vi "Parse Sysdef.vi"(0 "Device Reference in":T5 format="%.0x", 5 "error in (no error)":errorcluster) -> (6 "Status Config":T4 {"HWOut Dur Ref" format="%.0x"; "HWIn Dur Ref" format="%.0x"; "Error Data Ref" format="%.0x"}, 10 "HWIn BaseRate":i32, 12 "HWOut BaseRate":i32, 14 "Device Reference out":T5 format="%.0x", 15 "HWOutput Section Data":T6[](array[typedef]) {"Labels Settings"."Label" format="%.0o"}, 17 "HWInput Section Data":T6[](array[typedef]) {"Labels Settings"."Label" format="%.0o"}, 18 "Label Transfer Config":T1 {"Block Data Refs"."Data Reference" format="%.0x"}, 19 "error out":errorcluster)   [LabVIEW 2016, in "Ballard Arinc-429 Engine.lvlib"]
uses:
  Ballard Arinc-429 Engine.lvlib
  RT Controls/RT HW Channel.ctl
  RT Controls/RT Label Settings.ctl
  Shared/Controls and Global/Label.ctl
  Shared/Controls and Global/transferPeriod.ctl
  RT Controls/Driver Data.ctl
  RT Controls/RT Word Settings.ctl
  <vilib>/NI Veristand/Custom Device API/Block Data Reference.ctl
  <vilib>/NI Veristand/Custom Device API/Data Reference.ctl
  RT Controls/RT Param Setting.ctl
  Shared/Controls and Global/Start Bit.ctl
  Shared/Controls and Global/Number of Bits.ctl
  Shared/Controls and Global/TransferType.ctl
  <vilib>/NI Veristand/Custom Device API/Custom Device Item Ref.ctl
  RT Controls/Status Channels Config.ctl
  RT Controls/Label Transfer Config.ctl
  Shared/Controls and Global/Global.vi
  Shared/Ballard Arinc-429 Shared.lvlib
  <vilib>/NI Veristand/Custom Device API/Custom Device API.lvlib
  <vilib>/NI Veristand/Custom Device API/Get Item Property (Boolean).vi
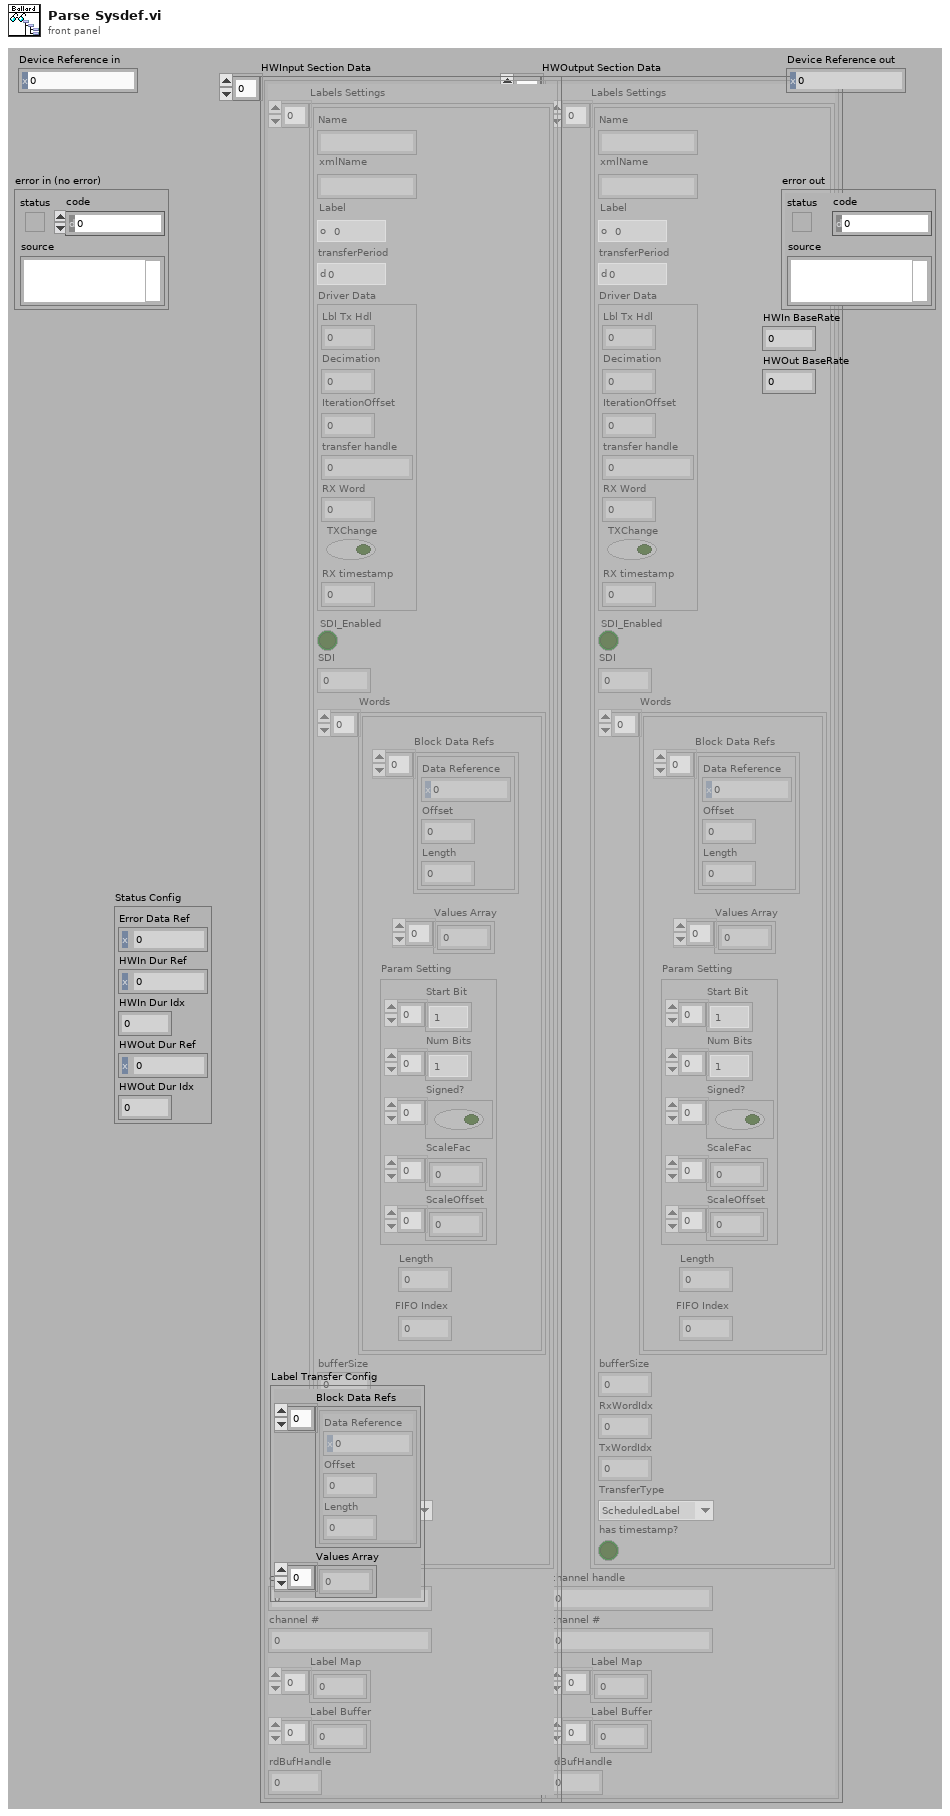
[diagram p1: front panel]
types:
  T1 = typedef "Ballard Arinc-429 Engine.lvlib/Label Transfer Config.ctl" = cluster{"Block Data Refs":T2[], "Values Array":dbl[]}
  T2 = typedef "Custom Device API.lvlib/Block Data Reference.ctl" = cluster{"Data Reference":T3, "Offset":u64, "Length":u64}
  T3 = typedef "Custom Device API.lvlib/Data Reference.ctl" = i32
  T4 = typedef "Ballard Arinc-429 Engine.lvlib/Status Channels Config.ctl" = cluster{"Error Data Ref":T3, "HWIn Dur Ref":T3, "HWIn Dur Idx":i32, "HWOut Dur Ref":T3, "HWOut Dur Idx":i32}
  T5 = typedef "Custom Device API.lvlib/Custom Device Item Ref.ctl" = u64
  T6 = typedef "Ballard Arinc-429 Engine.lvlib/RT HW Channel.ctl" = cluster{"Labels Settings":T7[], "channel handle":u32, "channel #":u16, "Label Map":i32[], "Label Buffer":u32[], "rdBufHandle":u32}
  T7 = typedef "Ballard Arinc-429 Engine.lvlib/RT Label Settings.ctl" = cluster{"Name":string, "xmlName":string, "Label":T8, "transferPeriod":T9, "Driver Data":T10, "SDI_Enabled":bool, "SDI":u8, "Words":T11[], "bufferSize":u32, "RxWordIdx":i32, "TxWordIdx":i32, "TransferType":T15, "has timestamp?":bool}
  T8 = typedef "Ballard Arinc-429 Shared.lvlib/Label.ctl" = u8
  T9 = typedef "Ballard Arinc-429 Shared.lvlib/transferPeriod.ctl" = u32
  T10 = typedef "Ballard Arinc-429 Engine.lvlib/Driver Data.ctl" = cluster{"Lbl Tx Hdl":u32, "Decimation":i32, "IterationOffset":i32, "transfer handle":u32, "RX Word":u32, "TXChange":bool, "RX timestamp":dbl}
  T11 = typedef "Ballard Arinc-429 Engine.lvlib/RT Word Settings.ctl" = cluster{"Block Data Refs":T2[], "Values Array":dbl[], "Length":i32, "FIFO Index":i32, "Param Setting":T12}
  T12 = typedef "Ballard Arinc-429 Engine.lvlib/RT Param Setting.ctl" = cluster{"Start Bit":T13[], "Num Bits":T14[], "Signed?":bool[], "ScaleFac":dbl[], "ScaleOffset":dbl[]}
  T13 = typedef "Ballard Arinc-429 Shared.lvlib/Start Bit.ctl" = i32
  T14 = typedef "Ballard Arinc-429 Shared.lvlib/Number of Bits.ctl" = i32
  T15 = typedef "Ballard Arinc-429 Shared.lvlib/TransferType.ctl" = enum16{"ScheduledLabel", "Acyclic", "Block", "Strobe"}
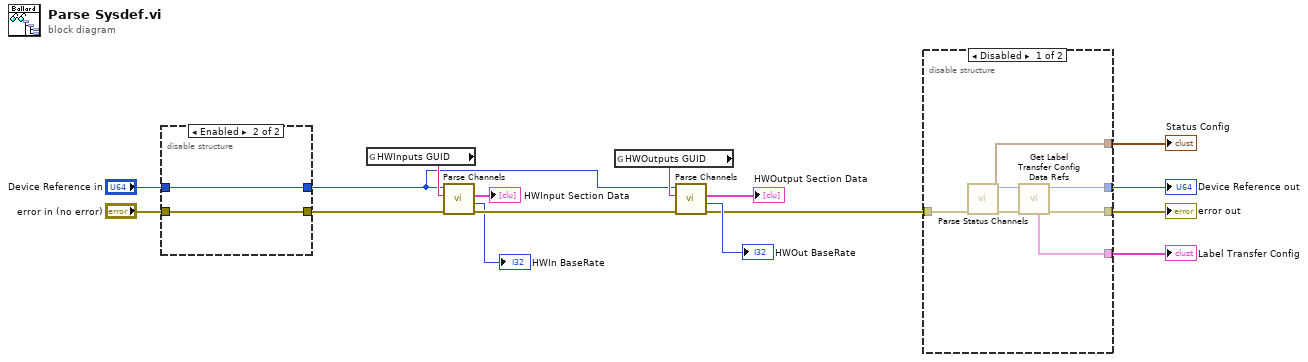
[diagram p0: block diagram]
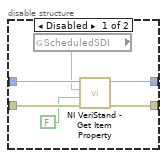
[diagram p3: hidden frame]
diagram:
  n1 = disable-structure shown="Enabled" {
    disable-tunnel: "Device Reference in" -> [w23 w25]
    disable-tunnel: [w22 w25] -> w1
    disable-tunnel: "error in (no error)" -> [w21 w24]
    disable-tunnel: [w20 w24] -> w2
    frame Disabled {
      n2 = global read "Global.vi" "ScheduledSDI"() -> (w18:string)
      n3 = call-poly <vilib>:"NI VeriStand - Get Item Property.vi"("error in (no error)"=w21, "Default Value"=FALSE, "Property Name"=w18, "Item Ref in"=w23) -> ("error out"=w20:errorcluster, "Value"=w19:bool, "Item Ref out"=w22:T5)  [unwired: 4 in, 1 out]
    }
    frame Enabled {
    }
  }
  n4 = global read "Global.vi" "HWInputs GUID"() -> (w14:string)
  n5 = call "Parse Channels.vi"("error in (no error)"=w2, "Section GUID"=w14, "Device Reference in"=w1) -> ("error out"=w15:errorcluster, "Section BaseRate"=→"HWIn BaseRate":i32, "Channel Data []"=→"HWInput Section Data":T6[])  [unwired: 6 in]
  n6 = global read "Global.vi" "HWOutputs GUID"() -> (w16:string)
  n7 = call "Parse Channels.vi"("error in (no error)"=w15, "Section GUID"=w16, "Device Reference in"=w1) -> ("error out"=w9:errorcluster, "Section BaseRate"=→"HWOut BaseRate":i32, "Channel Data []"=→"HWOutput Section Data":T6[])  [unwired: 6 in]
  n8 = disable-structure shown="Disabled" {
    disable-tunnel: w9 -> [w32 w33]
    disable-tunnel: [w31 _] -> w8
    disable-tunnel: [w28 w33] -> w7
    disable-tunnel: [w27 _] -> w6
    disable-tunnel: [w26 _] -> w5
    frame Disabled {
      n9 = call "Parse Status Channels.vi"("error in"=w32) -> ("error out"=w29:errorcluster, "Status Config"=w31:T4, "Device Ref out"=w30:T5)  [unwired: 8 in]
      n10 = call "Get Label Transfer Config Data Refs.vi"("error in"=w29, "Device Ref in"=w30) -> ("error out"=w28:errorcluster, "Device Ref out"=w27:T5, "Label Transfer Config"=w26:T1)  [unwired: 7 in]
    }
    frame Enabled {
    }
  }
  "Device Reference out" <- w6
  "error out" <- w7
  "Status Config" <- w8
  "Label Transfer Config" <- w5
